vi "SVG Parser.vi"(3 "error in (no error)":errorcluster, 5 "XML File Path":path) -> (0 "error out":errorcluster, 1 "Parsing Data":T2, 2 "Image Size":cluster{"Width":dbl, "Height":dbl})   [LabVIEW 2016]
doc: "This VI parses an SVG file using LabVIEW's built-in XML parser. It outputs the objects found in an SVG file as well as the canvas width and height."
uses:
  <vilib>/Analysis/Matrix/Datatypes/RealMatrix.ctl
  <vilib>/Analysis/Matrix/NI_Matrix.lvlib
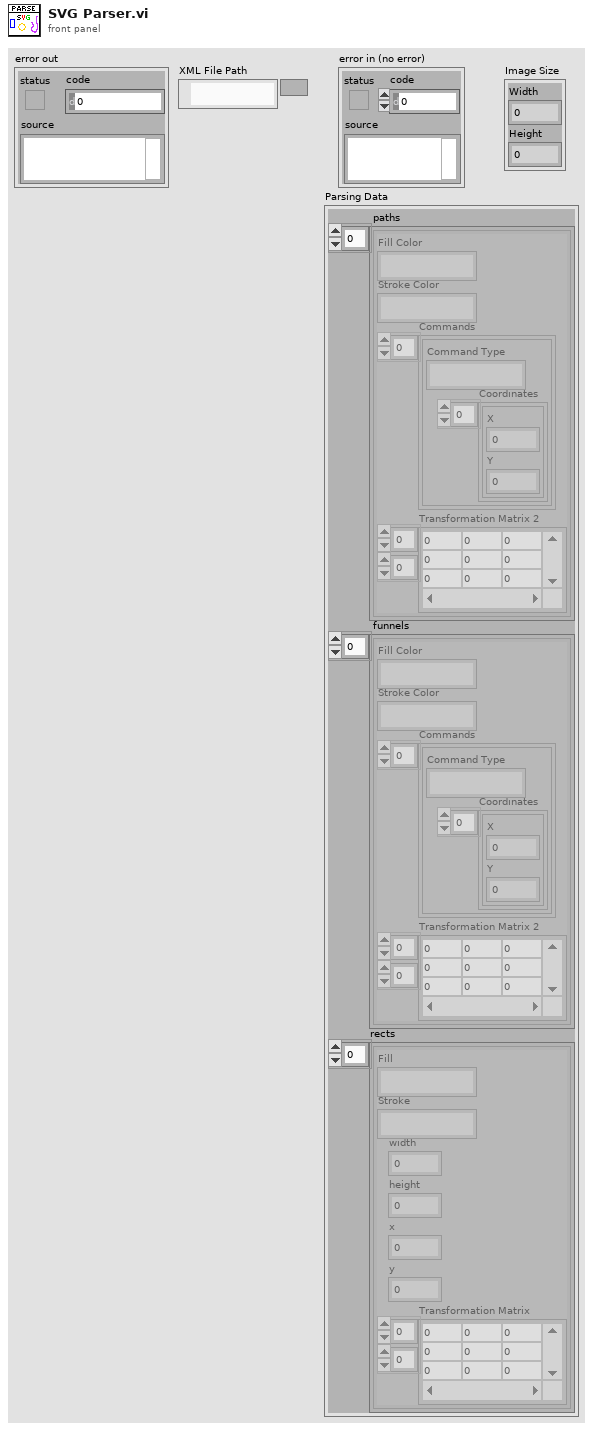
[diagram p1: front panel]
types:
  T1 = typedef "NI_Matrix.lvlib/RealMatrix.ctl" = dbl[][]
  T2 = cluster{" paths":cluster{"Fill Color":string, "Stroke Color":string, "Commands":cluster{"Command Type":string, "Coordinates":cluster{"X":dbl, "Y":dbl}[]}[], "Transformation Matrix 2":T1}[], " funnels":cluster{"Fill Color":string, "Stroke Color":string, "Commands":cluster{"Command Type":string, "Coordinates":cluster{"X":dbl, "Y":dbl}[]}[], "Transformation Matrix 2":T1}[], "rects":cluster{"Fill":string, "Stroke":string, "width":dbl, "height":dbl, "x":dbl, "y":dbl, "Transformation Matrix":T1}[]}
  T3 = cluster{"Fill Color":string, "Stroke Color":string, "Commands":cluster{"Command Type":string, "Coordinates":cluster{"X":dbl, "Y":dbl}[]}[], "Transformation Matrix 2":T1}[]
  T4 = cluster{"Fill":string, "Stroke":string, "width":dbl, "height":dbl, "x":dbl, "y":dbl, "Transformation Matrix":T1}[]
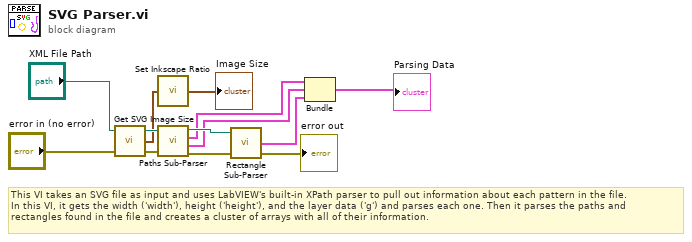
[diagram p0: block diagram]
diagram:
  # "This VI takes an SVG file as input and uses LabVIEW's built-in XPath parser to pull out information about each pattern in the file. \nIn this VI, it gets the width ('width'), height ('height'), and the layer data ('g') and parses each one. Then it parses the paths and \nrectangles found in the file and creates a cluster of arrays with all of their information."
  n1 = call "Get SVG Image Size.vi"("error in (no error)"="error in (no error)", "XML File Path In"="XML File Path") -> ("error out"=w10:errorcluster, "Image Size"=w6:cluster{"Width":dbl, "Height":dbl}, "XML File Path Out"=w11:path)  [unwired: 1 in]
  n2 = call "Set Inkscape Ratio.vi"("Image Size In"=w6) -> ("Image Size Out"=→"Image Size":cluster{"Width":dbl, "Height":dbl})
  n3 = call "Paths Sub-Parser.vi"("XML File Path In"=w11, "error in (no error)"=w10) -> ("XML File Path Out"=w8:path, "paths"=w5:T3, "funnels"=w4:T3, "error out"=w9:errorcluster)  [unwired: 1 in]
  n4 = call "Rectangle Sub-Parser.vi"("error in (no error)"=w9, "XML File Path In"=w8) -> ("error out"=→"error out":errorcluster, "rects"=w3:T4)  [unwired: 1 in, 1 out]
  n5 = Bundle("paths"=w5, "funnels"=w4, "rects"=w3) -> (→"Parsing Data":T2)  [unwired: 1 in]
